vi "PH_TKTDS-30xx.Configure Acquisition.vi"(0 "i ref in":refnum<vi>, 2 "Acquisition Configuration":T1={"Time base"=2e-07, "Record Length"=10000, "Start Time"=0.0, "Type"=0, "Continuous"=FALSE} {"Start Time" format="%#_12p"; "Record Length" items=["500"=500, "10000"=10000]; "Time base" items=["2ns"=2e-09, "4ns"=4e-09, "10ns"=1e-08, "20ns"=2e-08, "40ns"=4e-08, "100ns"=1e-07, "200ns"=2e-07, "400ns"=4e-07, "1µs"=1e-06, "2µs"=2e-06, "4µs"=4e-06, "10µs"=1e-05, "20µs"=2e-05, "40µs"=4e-05, "100µs"=0.0001, "200µs"=0.0002, "400µs"=0.0004, "1ms"=0.001, "2ms"=0.002, "10ms"=0.01, "20ms"=0.02, "40ms"=0.04, "100ms"=0.1, "200ms"=0.2, "400ms"=0.4, "1s"=1.0, "2s"=2.0, "4s"=4.0, "10s"=10.0]}, 5 "error IO":errorcluster) -> (14 "i ref out":refnum<vi>, 19 "error out":errorcluster)   [LabVIEW 2014, in "PH_TKTDS-30xx.lvlib"]
doc: "If the connection is established, the acquisition configuration is set and written to own attributes as well as the errors."
uses:
  PH_TKTDS-30xx.lvlib
  PH_TKTDS-30xx.Acquisition Config.ctl
  instr.lib/TKDS3032-PHELIX/tktds3032-PHELIX - Driver np.lvlib
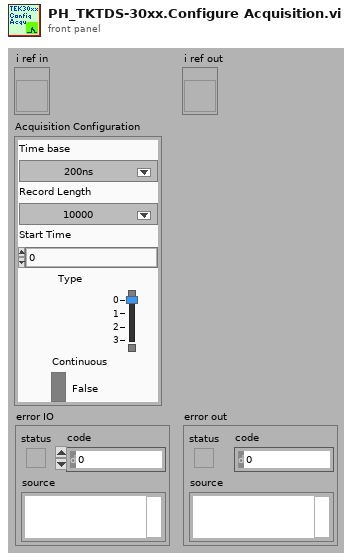
[diagram p1: front panel]
types:
  T1 = typedef "PH_TKTDS-30xx.lvlib/PH_TKTDS-30xx.Acquisition Config.ctl" = cluster{"Time base":dbl, "Record Length":u16, "Start Time":dbl, "Type":i32, "Continuous":bool}
  T2 = typedef "PH_TKTDS-30xx.lvlib/PH_TKTDS-30xx.i attribute.ctl" = cluster{"Default VISA Resource":string, "VISA Resource Name":refnum<visa-resource-name>, "Revision":cluster{"Instrument Driver":string, "Instrument Firmware":string}, "Selftest":cluster{"Result":u32, "Message":string}, "Channels":T3[], "Trigger Configuration":T5, "Acquisition Configuration":T1, "Fetched Waveforms":T6[], "GUI Refs":T7, "State":T8, "Error Message":string, "Allow Prdc Loop?":bool}
  T3 = typedef "PH_TKTDS-30xx.lvlib/PH_TKTDS-30xx.Channel Config.ctl" = cluster{"Channel Name":string, "Input Impedance":string, "Max Input Frequency":string, "Vertical Coupling":i32, "Channel Enabled":bool, "Probe Attenuation":dbl, "Vertical Range":dbl, "Vertical Offset":dbl, "Waveform Limits":T4}
  T4 = typedef "PH_TKTDS-30xx.lvlib/PH_TKTDS-30xx.Waveform Limits.ctl" = cluster{"Start":i32, "End":i32}
  T5 = typedef "PH_TKTDS-30xx.lvlib/PH_TKTDS-30xx.Trigger Config.ctl" = cluster{"Source":string, "Slope":i32, "Level [V]":dbl}
  T6 = typedef "PH_TKTDS-30xx.lvlib/PH_TKTDS-30xx.fetched Waveform.ctl" = cluster{"Source":string, "Actual Points":u32, "Initial X":dbl, "X Increment":dbl, "Waveform Array":dbl[]}
  T7 = typedef "PH_TKTDS-30xx.lvlib/PH_TKTDS-30xx.GUI Refs.ctl" = cluster{"Trigger":refnum<vi>, "Acquisition":refnum<vi>, "State":refnum<vi>, "Delete":refnum<vi>, "Channel to be positioned":refnum<vi>, "Postion":refnum<vi>, "Display Intensity":refnum<vi>, "VISA Resource":refnum<vi>, "Channels":refnum<vi>[], "Graphs":refnum<vi>[]}
  T8 = typedef "PH_StatusHandler.lvlib/PH_StatusHandler.Status.ctl" = i16
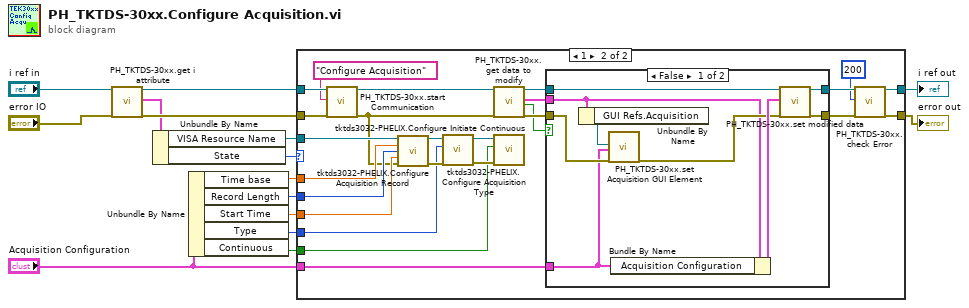
[diagram p0: block diagram]
diagram:
  n1 = call "PH_TKTDS-30xx.get i attribute.vi"("i ref in"="i ref in", "error in (no error)"="error IO") -> ("i ref out"=w10:refnum<vi>, "i attribute"=w12:T2, "error out"=w14:errorcluster)  [unwired: 15 in]
  n2 = Unbundle By Name(w12) -> ("VISA Resource Name"=w13:refnum<visa-resource-name>, "State"=w2:T8)
  n3 = Unbundle By Name("Acquisition Configuration") -> ("Time base"=w7:dbl, "Record Length"=w6:u16, "Start Time"=w5:dbl, "Type"=w4:i32, "Continuous"=w3:bool)
  n4 = case shown="1" w2 {
    tunnel: w10 -> [w17 w24]
    tunnel: w13 -> [_ w34]
    tunnel: [w16 w25] -> w8
    tunnel: w14 -> [w16 w37]
    tunnel: [w17 w21] -> w15
    tunnel: w7 -> [_ w31]
    tunnel: w6 -> [_ w30]
    tunnel: w5 -> [_ w29]
    tunnel: w4 -> [_ w28]
    tunnel: w3 -> [_ w27]
    tunnel: "Acquisition Configuration" -> [_ w18]
    frame Default {
    }
    frame 1 {
      n5 = call "PH_TKTDS-30xx.start Communication.vi"("i ref in"=w24, "Action"="Configure Acquisition", "error in"=w37) -> ("i ref out"=w23:refnum<vi>, "error out"=w26:errorcluster)  [unwired: 15 in]
      n6 = call "tktds3032-PHELIX.Configure Acquisition Record.vi"("VISA Resource Name"=w34, "Time base"=w31, "Record Length"=w30, "Acquisition Start Time (0.0 s)"=w29, "error in (no error)"=w26) -> ("VISA Resource Name Out"=w33:refnum<visa-resource-name>, "error out"=w36:errorcluster)  [unwired: 9 in]
      n7 = call "tktds3032-PHELIX.Configure Acquisition Type.vi"("error in (no error)"=w36, "Acquisition Type (0:Sample)"=w28, "VISA Resource Name"=w33) -> ("error out"=w35:errorcluster, "VISA Resource Name Out"=w32:refnum<visa-resource-name>)  [unwired: 7 in]
      n8 = call "PH_TKTDS-30xx.get data to modify.vi"("i ref in"=w23, "error in (no error)"=w26) -> ("i ref out"=w40:refnum<vi>, "i attribute"=w38:T2, "timed out"=w39:bool, "error out"=w41:errorcluster)  [unwired: 14 in]
      n9 = call "tktds3032-PHELIX.Configure Initiate Continuous.vi"("error in (no error)"=w35, "Continuous Acquisition (False)"=w27, "VISA Resource Name"=w32) -> ()  [unwired: 7 in, 2 out]
      n10 = case shown="False" w39 {
        tunnel: [w51 w52] -> w42
        tunnel: w41 -> [w50 w52]
        tunnel: w40 -> [w49 w53]
        tunnel: [w48 w53] -> w22
        tunnel: w38 -> [w45 _]
        tunnel: w18 -> [w43 _]
        frame False {
          n11 = Unbundle By Name(w45) -> ("GUI Refs.Acquisition"=w44:refnum<vi>)
          n12 = call "PH_TKTDS-30xx.set Acquisition GUI Element.vi"("Ref Acquisition Config"=w44, "Acqu Config"=w43, "error in"=w50) -> ("error out"=w46:errorcluster)  [unwired: 16 in]
          n13 = Bundle By Name(cluster=w45, "Acquisition Configuration"=w43) -> (w47:T2)
          n14 = call "PH_TKTDS-30xx.set modified data.vi"("i ref in"=w49, "i attribute"=w47, "error in (no error)"=w46) -> ("i ref out"=w48:refnum<vi>, "error out"=w51:errorcluster)  [unwired: 15 in]
        }
        frame True {
        }
      }
      n15 = call "PH_TKTDS-30xx.check Error.vi"("i ref in"=w22, "Waiting Time [ms]"=u32 200, "error in"=w42) -> ("i ref out"=w21:refnum<vi>, "error out"=w25:errorcluster)  [unwired: 15 in]
    }
  }
  "i ref out" <- w15
  "error out" <- w8
